vi "AddTestMethod_CreateNewWizard_GetWeight.vi"(11 "Wizard":T1) -> (3 "Weight":i32)   [LabVIEW 2013]
uses:
  <resource>/Framework/Providers/API/ItemRef.ctl
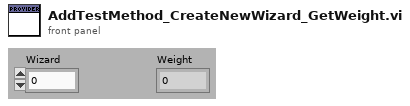
[diagram p1: front panel]
types:
  T1 = typedef "ItemRef.ctl" = u64
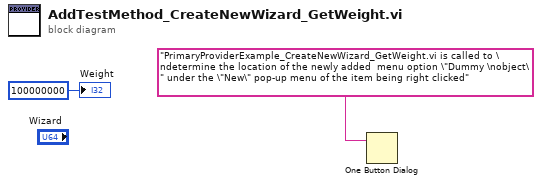
[diagram p0: block diagram]
diagram:
  n1 = One Button Dialog(message="PrimaryProviderExample_CreateNewWizard_GetWeight.vi is called to \ndetermine the location of the newly added  menu option \"Dummy \nobject\" under the \"New\" pop-up menu of the item being right clicked") -> ()  [unwired: 1 in, 1 out]
  "Weight" <- 100000000 ("Weight")
